vi "zadanie2.vi"() -> ()   [LabVIEW 2012]
panel:
  out "Wykres zmiany temperatury pacjenta od 01.12.2020 do 13.12.2020":dbl[](graph)
  # "Program pokazuje wykres temperatury pacjenta od 01.12.20202 do 13.12.2020"
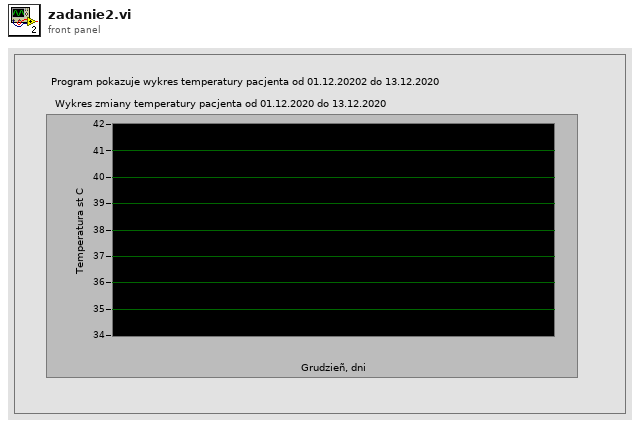
[diagram p1: front panel]
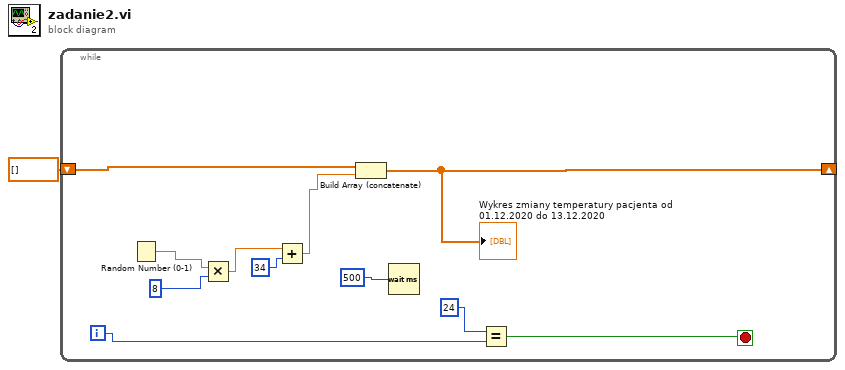
[diagram p0: block diagram]
diagram:
  n1 = while {
    shift-right: [w6] -> _
    shift-left: dbl[] [] -> [w12]
    i -> [w2]
    stop <- w4 stop-if-true
    n2 = Random Number (0-1)() -> (number: 0 to 1=w8:dbl)
    n3 = Multiply(x=w8, y=8) -> (x*y=w10:dbl)
    n4 = Add(x=w10, y=34) -> (x+y=w7:dbl)
    n5 = Build Array (concatenate)(w12, w7) -> (w6:dbl[])
    "Wykres zmiany temperatury pacjenta od 01.12.2020 do 13.12.2020" <- w6
    n6 = Wait (ms)(milliseconds to wait=500) -> ()  [unwired: 1 out]
    n7 = Equal?(x=24, y=w2) -> (x = y?=w4:bool)
  }
